vi "Get_Aug_Config.vi"(11 "Aug Factor":enum16{"2x", "4x", "8x"}(ring)) -> (3 "Aug_Config":cluster{"Flip?":bool, "Rotation":T1}[](array[cluster]))   [LabVIEW 2020]
uses:
  Controls/Aug_Rotation.ctl
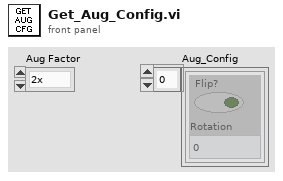
[diagram p1: front panel]
types:
  T1 = typedef "Aug_Rotation.ctl" = enum16{"0", "90", "180", "270"}
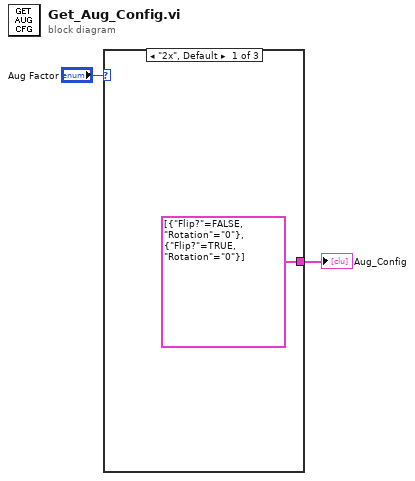
[diagram p0: block diagram]
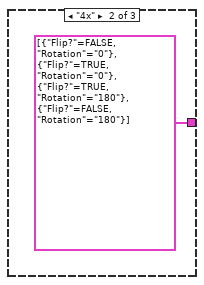
[diagram p2: hidden frame]
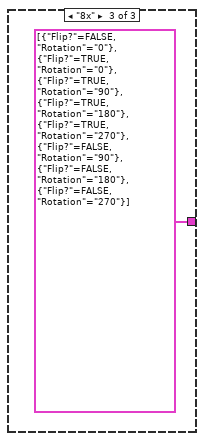
[diagram p3: hidden frame]
diagram:
  n1 = case shown="\"2x\", Default" "Aug Factor" {
    tunnel: [cluster{"Flip?":bool, "Rotation":T1}[] [{"Flip?"=FALSE, "Rotation"=enum."0"}, {"Flip?"=TRUE, "Rotation"=enum."0"}] ("Cluster") cluster{"Flip?":bool, "Rotation":T1}[] [{"Flip?"=FALSE, "Rotation"=enum."0"}, {"Flip?"=TRUE, "Rotation"=enum."0"}, {"Flip?"=TRUE, "Rotation"=enum."180"}, {"Flip?"=FALSE, "Rotation"=enum."180"}] ("Cluster") cluster{"Flip?":bool, "Rotation":T1}[] [{"Flip?"=FALSE, "Rotation"=enum."0"}, {"Flip?"=TRUE, "Rotation"=enum."0"}, {"Flip?"=TRUE, "Rotation"=enum."90"}, {"Flip?"=TRUE, "Rotation"=enum."180"}, {"Flip?"=TRUE, "Rotation"=enum."270"}, {"Flip?"=FALSE, "Rotation"=enum."90"}, {"Flip?"=FALSE, "Rotation"=enum."180"}, {"Flip?"=FALSE, "Rotation"=enum."270"}] ("Cluster")] -> w2
    frame "2x", Default {
    }
    frame "4x" {
    }
    frame "8x" {
    }
  }
  "Aug_Config" <- w2
